vi "题目一.vi"() -> ()   [LabVIEW 2017]
panel:
  out "波形图表":dbl(graph)
  in  "滑动杆":i32(slide) scale=0.0..10.0
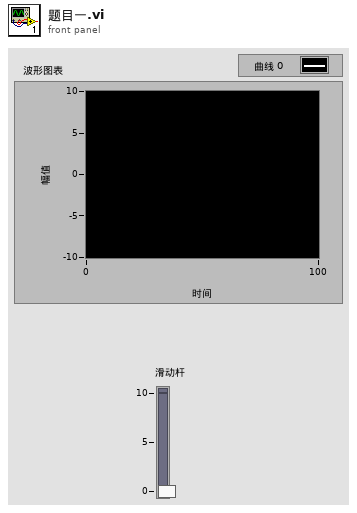
[diagram p1: front panel]
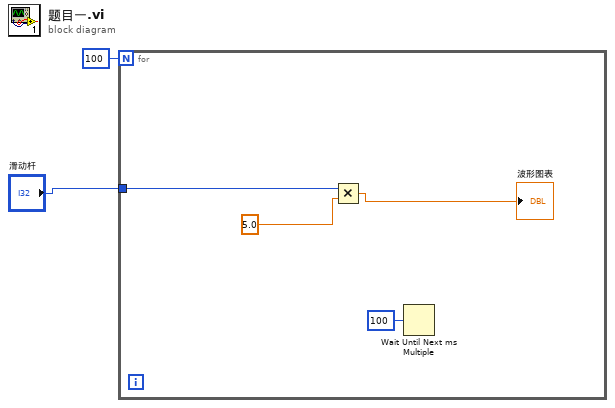
[diagram p0: block diagram]
diagram:
  n1 = for {
    N: 100 -> [_]
    tunnel: "滑动杆" -> [w3]
    n2 = Multiply(x=w3, y=5.0) -> (x*y=→"波形图表":dbl)
    n3 = Wait Until Next ms Multiple(millisecond multiple=u32 100 ("毫秒倍数")) -> ()  [unwired: 1 out]
  }
